vi "autonomous pure pursuit.vi"(10 "Waypoint Data":cluster{"Waypoints":dbl[][], "Reverse?":bool}={"Waypoints"=[[0.0, 0.0], [2.0, 30000.0], [20000.0, 60000.0]], "Reverse?"=FALSE}, 11 "Button":bool) -> ()   [LabVIEW 2018]
uses:
  path data.ctl
  <vilib>/Rock Robotics/WPI/DriverStation/WPI_DriverStationDerivedRobotMode.ctl
  TypeDefs/typedef_enum_Refnums.ctl
  <vilib>/Rock Robotics/WPI/Utilities/WPI_GetSetVariantRefNum.vi
  <vilib>/ptbypt/NI_PtbyPt.lvlib
  <vilib>/Rock Robotics/WPI/RobotDrive/WPI_RobotDriveArcadeDrive_Standard(NoSaturation).vi
  <vilib>/Rock Robotics/Network Tables/NT Write Boolean.vi
panel:
  in  "Path Data":T1={"Path"=[], "Target Velocities"=[], "Robot Location"=[0.0, 0.0], "Relative Robot Angle (rad)"=0.0, "Curvature"=0.0, "Lookahead Point"=[0.0, 0.0], "Lookahead Index"=0.0, "Closest Point"=[0.0, 0.0], "Closest Point Index"=0, "Left Velocity"=0.0, "Right Velocity"=0.0, "Left Encoder Vel"=0, "Right Encoder Vel"=0, "Left Encoder Pos"=0, "Right Encoder Pos"=0, "Inital Robot Angle (deg)"=0.0}
  in  "Diagnostic?":bool=TRUE
  in  "Tuning":T2={"Kv Left"=0.00023, "Kv Right"=0.00023, "Kp Left"=0.0001, "Kp Right"=0.0001}
  out "Loop Time":u32=44680
  out "Exp. Curvature":dbl[](graph)=[0.0, 1.4034333257619034e-07, 3.165606565156983e-07, 5.735690112841907e-07, 9.783335869805837e-07, 1.6388561568734111e-06, 2.7401762932584762e-06, 4.610837725094686e-06, 7.868434900770625e-06, 1.3752057162216792e-05, 2.4965310123263664e-05, 4.7908917652252264e-05, 6.401235309575295e-05, 3.360888592844542e-05, 1.8452253376050564e-05, 1.0514808142316512e-05, 6.145592499109037e-06, 3.650831804118769e-06, 2.191028177213592e-06, 1.3231905148774929e-06, 8.018237673268363e-07, 4.861886501530978e-07, 2.9338742319180646e-07, 1.7372213438406245e-07, 9.640327443482198e-08, 4.0874668672438526e-08, 0.0]
  out "Curvature":dbl(graph)
  out "Target Velocities":cluster{dbl, dbl}(graph)={850.0, 850.0}
  in  "Lookahead Distance":dbl=5000.0 format="%#_13g"
  out "Path":T3(graph)=[{"Smooth Path"=[0.0, 3.9831976339745525, 8.918786774310743, 15.996756278926227, 26.94310215462526, 44.45175679243214, 72.85576199340136, 119.21333672590853, 195.06952147459873, 319.3449114169336, 523.0654465520985, 857.1178508590853, 1404.971654642396, 2303.5684955547395, 3415.918100969553, 4658.468244850319, 5980.216850342943, 7349.961644912561, 8748.499353660785, 10163.825114581763, 11588.130666803412, 13015.85297046767, 14442.283167634836, 15862.389189218296, 17269.55815292861, 18653.942887255045, 20000.0], "Smooth Path"=[0.0, 2604.6593521886216, 5208.4834070465695, 7810.428161388078, 10408.979451847843, 13001.776283234469, 15585.016727668002, 18152.511956181766, 20694.135215630122, 23193.291890529486, 25622.77148689383, 27937.944042539046, 30065.60256829882, 32209.66168633789, 34363.622817575204, 36523.46279208931, 38686.62801955882, 40851.39631476969, 43016.44613594504, 45180.526806154805, 47342.144596973565, 49499.19086028001, 51648.41344856078, 53784.60445996854, 55899.29829439407, 57978.65493411005, 60000.0]}, {"Smooth Path"=[-155.34781165121697, -32.634161371312175], "Smooth Path"=[-10126.308473842537, -2127.2496942088364]}, {"Smooth Path"=[0.0], "Smooth Path"=[0.0]}, {"Smooth Path"=[0.0, -155.34781165121697], "Smooth Path"=[0.0, -10126.308473842537]}]
  in  "Config":T4={"Path"={"Spacing"=2608.0, "Smooth Weight"=0.8, "Tolerance"=0.01}, "Kinematics"={"Max Vel"=850.0, "Max Accel"=200.0, "Curvature Const"=1.0}}
  in  "Track Width":dbl=13000.0 format="%#_13g"
  out "Right Output":dbl=0.24650000000000002
  out "Left Output":dbl=0.23800000000000002
  out "Left Velocity":T5(graph)={"Quadrature Velocity"=0, "Left Velocity"=850.0}
  out "Right Velocity":T6(graph)={"Quadrature Velocity"=0, "Right Velocity"=850.0}
  out "Robot Angle":dbl=-0.87890625
  out "Curvature":dbl
  out "Robot Location":dbl[](array[numeric])=[-155.34781165121697, -10126.308473842537]
  out "Right Velocity":dbl=850.0
  out "Left Velocity":dbl=850.0
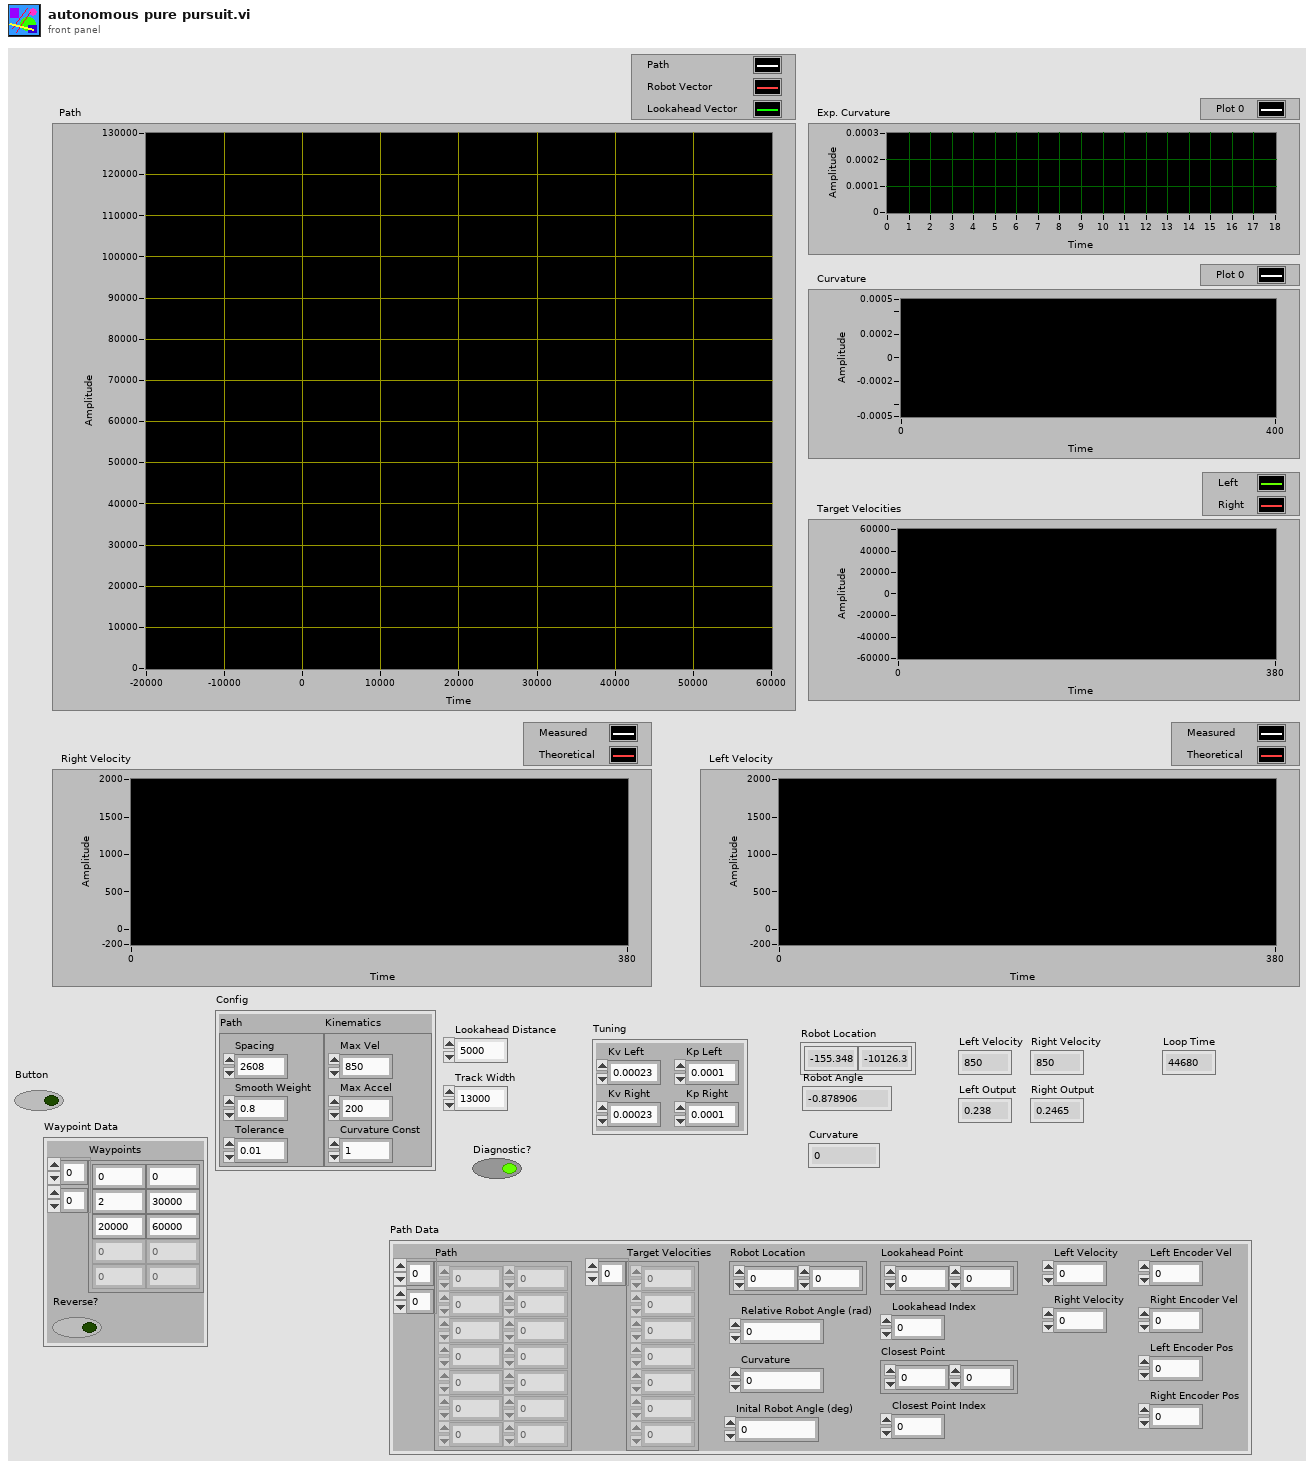
[diagram p1: front panel]
types:
  T1 = typedef "path data.ctl" = cluster{"Path":dbl[][], "Target Velocities":dbl[], "Robot Location":dbl[], "Relative Robot Angle (rad)":dbl, "Curvature":dbl, "Lookahead Point":dbl[], "Lookahead Index":dbl, "Closest Point":dbl[], "Closest Point Index":i32, "Left Velocity":dbl, "Right Velocity":dbl, "Left Encoder Vel":i32, "Right Encoder Vel":i32, "Left Encoder Pos":i32, "Right Encoder Pos":i32, "Inital Robot Angle (deg)":dbl}
  T2 = cluster{"Kv Left":dbl, "Kv Right":dbl, "Kp Left":dbl, "Kp Right":dbl}
  T3 = cluster{"Smooth Path":dbl[], "Smooth Path":dbl[]}[]
  T4 = cluster{"Path":cluster{"Spacing":dbl, "Smooth Weight":dbl, "Tolerance":dbl}, "Kinematics":cluster{"Max Vel":dbl, "Max Accel":dbl, "Curvature Const":dbl}}
  T5 = cluster{"Quadrature Velocity":i32, "Left Velocity":dbl}
  T6 = cluster{"Quadrature Velocity":i32, "Right Velocity":dbl}
  T7 = typedef "WPI_DriverStationDerivedRobotMode.ctl" = enum16{"Init", "Execute", "Stop"}
  T8 = typedef "typedef_enum_Refnums.ctl" = enum16{"Ball_Encoder", "Ball_Motor", "Camera", "Linefollow_3", "Linefollow_2", "Linefollow_1", "Gyro", "Hatch_Solenoid", "Climb_Back_Solenoid", "Arm_Encoder", "Arm_Motor", "Lift_Encoder", "Drive", "Drive_Motor_R", "Drive_Motor_L", "Drive_Encoder_R", "Drive_Encoder_L", "Joy_R", "Joy_L", "Wrist_Motor", "Wrist_Encoder", "Climb Upper Limit", "Climb Lower Limit ", "Climb_Front_Motor"}
  T9 = typedef "Teleop Data Cluster.ctl" = cluster{"Drive Forward Input ":dbl, "Drive Twist Input":dbl, "Drive Output":dbl, "Drivetwist Output":dbl, "Left Joystick Buttons":bool[], "Left Joystick Axis":dbl[], "Right Joystick Axis":dbl[], "Right Joystick Button":bool[], "Arm Encoder":dbl, "Left Drive Encoder":dbl, "Right Drive Encoder":dbl, "Gyro Angle ":dbl, "Arm Joystick Output  ":dbl, "Line Follower L, C, R ":bool[], "Line follow?":bool, " Climb Solenoid":bool, "Wrist Encoder Count":dbl, "Wrist Joystick Output":dbl, "Ball Encoder Count":dbl, "Ball Output":dbl, "Climb Encoder":dbl, "Climb Motor Output":dbl, " Hatch Solenoid":bool, "Arm Setpoint ":dbl, "Wrist Setpoint ":dbl, "Arm Joystick Enabled?":bool, "Wrist Joystick Enabled":bool, "Vision String":string}
  T10 = typedef "WPI_RobotDriveDevRef.ctl" = cluster{"DevStatus":errorcluster, "Motors[]":T11[], "Square Inputs":bool, "Max Output":dbl}
  T11 = typedef "WPI_MotorControlDeviceRef.ctl" = cluster{"DeviceStatus":errorcluster, "Type":T12, "PWM":cluster{"PWM Channel":T13, "DeadBand":T14}, "CAN":cluster{"Device Number":u8, "SetOutput VI Ref":variant, "GetOutput VI Ref":variant, "Enable VI Ref":variant, "Disable VI Ref":variant, "Data":variant}, "Invert":bool, "DIO PWM":cluster{"PWM \"Enable\" Channel":T13, "DIOChannel":T15, "PWM Rate":dbl}}
  T12 = typedef "WPI_MotorControlType.ctl" = enum16{"PWM", "CAN", "DIO PWM"}
  T13 = typedef "FPGA_DIOPWMChannel.ctl" = enum8{"PWM 0", "PWM 1", "PWM 2", "PWM 3", "PWM 4", "PWM 5", "PWM 6", "PWM 7", "PWM 8", "PWM 9", "PWM MXP 0", "PWM MXP 1", "PWM MXP 2", "PWM MXP 3", "PWM MXP 4", "PWM MXP 5", "PWM MXP 6", "PWM MXP 7", "PWM MXP 8", "PWM MXP 9", "Invalid"}
  T14 = typedef "WPI_PWMDeadband.ctl" = cluster{"Name":string, "maxPositivePwm":i32, "minPositivePwm":i32, "centerPwm":i32, "maxNegativePwm":i32, "minNegativePwm":i32, "angularRange":u16}
  T15 = typedef "FPGA_DIOChannel.ctl" = enum8{"DIO 0", "DIO 1", "DIO 2", "DIO 3", "DIO 4", "DIO 5", "DIO 6", "DIO 7", "DIO 8", "DIO 9", "DIO MXP 0", "DIO MXP 1", "DIO MXP 2", "DIO MXP 3", "DIO MXP 4", "DIO MXP 5", "DIO MXP 6", "DIO MXP 7", "DIO MXP 8", "DIO MXP 9", "DIO MXP 10", "DIO MXP 11", "DIO MXP 12", "DIO MXP 13", "DIO MXP 14", "DIO MXP 15", "SPI Port CS1", "SPI Port CS2", "SPI Port CS3", "SPI Port MISO", "SPI Port MOSI", "Invalid"}
  T16 = typedef "CTRE_PigeonIMU_DeviceRef.ctl" = cluster{"DeviceStatus":errorcluster, "Device Number":u8, "Type":T17, "Device ID":u32, "Handle":u64, "UsageFrame":u32, "Library Path":path}
  T17 = typedef "CTRE_PigeonIMU_ConnectionType.ctl" = u32
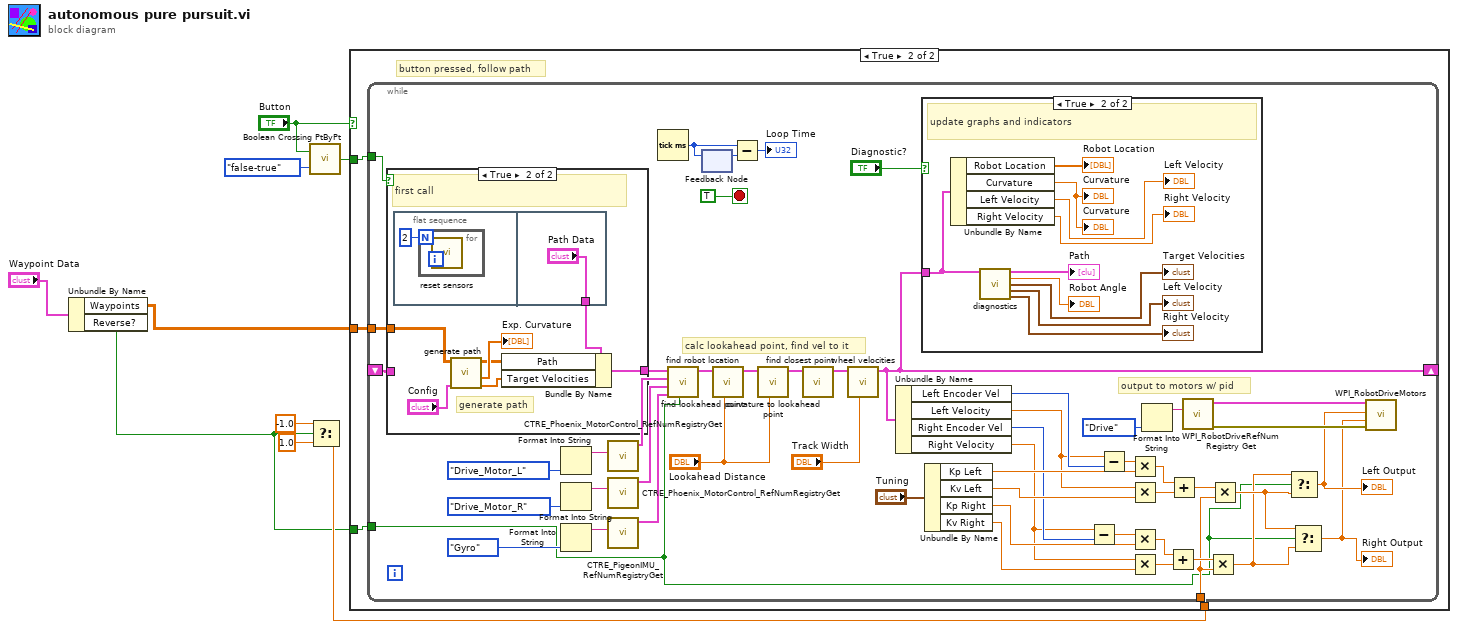
[diagram p0: block diagram]
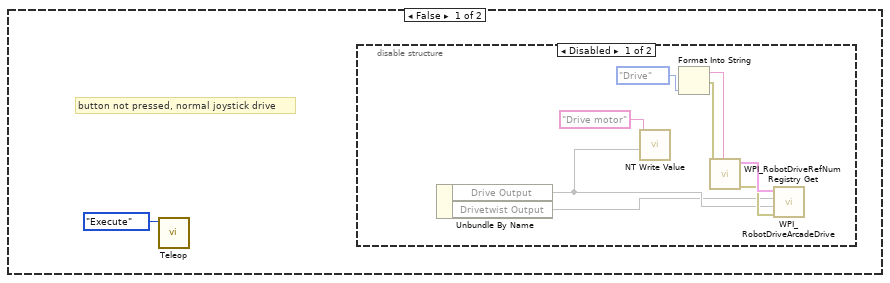
[diagram p2: hidden frame]
diagram:
  n1 = Unbundle By Name("Waypoint Data") -> ("Waypoints"=w2:dbl[][], "Reverse?"=w1:bool)
  n2 = call <vilib>:"Boolean Crossing PtByPt.vi"("direction"=enum16{"either", "false-true", "true-false"}."false-true", "input"="Button") -> ("crossing"=w7:bool)  [unwired: 1 in]
  n3 = Select(t=-1.0, s=w1, f=1.0) -> (s? t:f=w4:dbl)
  n4 = case shown="True" "Button" {
    tunnel: w7 -> [_ w23]
    tunnel: w4 -> [_ w22]
    tunnel: w1 -> [_ w21]
    tunnel: w2 -> [_ w20]
    frame False {
      # "button not pressed, normal joystick drive"
      n5 = call "Teleop.vi"("Call Context"=WPI_DriverStationDerivedRobotMode."Execute") -> ()  [unwired: 11 in]
      n6 = disable-structure shown="Disabled" {
        frame Disabled {
          n7 = Unbundle By Name() -> (w13:T9, "Drive Output"=w14, "Drivetwist Output"=w11)
          n8 = call-poly <vilib>:"NT Write Value.vi"("Boolean"=w14, "Name"="Drive motor") -> ()  [unwired: 9 in, 1 out]
          n9 = Format Into String(typedef_enum_Refnums."Drive" ("RefNums")) -> (resulting string=w18:string, error out=w16:errorcluster)  [unwired: 3 in]
          n10 = call <vilib>:"WPI_RobotDriveRefNum Registry Get.vi"("error in (no error)"=w16, "refnum name"=w18) -> ("error out"=w15:errorcluster, "RobotDriveDevRef"=w19:T10)  [unwired: 8 in]
          n11 = call-poly <vilib>:"WPI_RobotDriveArcadeDrive.vi"("error in (no error)"=w15, "Y axis value"=w14, "X axis value"=w11, "RobotDriveDevRef"=w19) -> ()  [unwired: 5 in, 3 out]
        }
        frame Enabled {
        }
      }
    }
    frame True {
      # "button pressed, follow path"
      n12 = while {
        tunnel: w23 -> [w39]
        shift-right: [w41] -> _
        shift-left: _ -> [w50]
        tunnel: w22 -> [w30]
        tunnel: w21 -> [w25]
        tunnel: w20 -> [w24]
        stop <- TRUE stop-if-true
        # "calc lookahead point, find vel to it"
        # "output to motors w/ pid"
        n13 = case shown="True" w39 {
          tunnel: [w86 w89] -> w40
          tunnel: w50 -> [w86 _]
          tunnel: w24 -> [_ w88]
          frame False {
          }
          frame True {
            # "generate path"
            # "first call"
            n14 = flat-sequence {
              tunnel: ["Path Data"] -> w87
              frame #0 {
                n15 = for {
                  N: 2 -> [_]
                  n16 = call "reset sensors.vi"() -> ()  [unwired: 12 in]
                }
              }
              frame #1 {
              }
            }
            n17 = call "generate path.vi"("Config"="Config", "Waypoints"=w88) -> ("Target Velocities"=w90:dbl[], "Curvatures"=→"Exp. Curvature":dbl[], "Smooth Path"=w91:dbl[][])  [unwired: 4 in, 3 out]
            n18 = Bundle By Name(cluster=w87, "Path"=w91, "Target Velocities"=w90) -> (w89:T1)
          }
        }
        n19 = Format Into String(typedef_enum_Refnums."Drive_Motor_L" ("RefNums")) -> (resulting string=w35:string)  [unwired: 3 in, 1 out]
        n20 = Format Into String(typedef_enum_Refnums."Drive_Motor_R" ("RefNums")) -> (resulting string=w34:string)  [unwired: 3 in, 1 out]
        n21 = Format Into String(typedef_enum_Refnums."Gyro" ("RefNums")) -> (resulting string=w33:string)  [unwired: 3 in, 1 out]
        n22 = call <vilib>:"CTRE_Phoenix_MotorControl_RefNumRegistryGet.vi"("refnum name"=w35) -> ("PhoenixMotorControlDevRef"=w46:T11)  [unwired: 9 in, 1 out]
        n23 = call <vilib>:"CTRE_Phoenix_MotorControl_RefNumRegistryGet.vi"("refnum name"=w34) -> ("PhoenixMotorControlDevRef"=w47:T11)  [unwired: 9 in, 1 out]
        n24 = call <vilib>:"CTRE_PigeonIMU_RefNumRegistryGet.vi"("refnum name"=w33) -> ("PigeonIMUDevRef"=w48:T16)  [unwired: 9 in, 1 out]
        n25 = Tick Count (ms)() -> (millisecond timer value=w67:u32)
        n26 = call "find robot location.vi"("Reverse?"=w25, "Pigeon Reference"=w48, "Right Encoder Reference"=w47, "Left Encoder Reference"=w46, "Path Data"=w40) -> ("Path Data"=w49:T1)  [unwired: 6 in]
        n27 = feedback-in #1(w67) -> ()
        n28 = feedback #1() -> (w66:u32)  [unwired: 1 in]
        n29 = call "find lookahead point.vi"("Lookahead Distance"="Lookahead Distance", "Path Data"=w49) -> ("Path Data"=w53:T1)  [unwired: 9 in]
        n30 = Subtract(x=w67, y=w66) -> (x-y=→"Loop Time":u32)
        n31 = call "curvature to lookahead point.vi"("Lookahead Distance"="Lookahead Distance", "Path Data"=w53) -> ("Path Data"=w52:T1)  [unwired: 9 in]
        n32 = call "find closest point.vi"("Path Data"=w52) -> ("Path Data"=w51:T1)  [unwired: 10 in]
        n33 = call "wheel velocities.vi"("Track Width"="Track Width", "Path Data"=w51) -> ("Path Data"=w41:T1)  [unwired: 9 in]
        n34 = Unbundle By Name(w41) -> ("Left Encoder Vel"=w45:i32, "Left Velocity"=w44:dbl, "Right Encoder Vel"=w43:i32, "Right Velocity"=w42:dbl)
        n35 = case shown="True" "Diagnostic?" {
          tunnel: w41 -> [_ w76]
          frame False {
          }
          frame True {
            # "update graphs and indicators"
            n36 = Unbundle By Name(w76) -> ("Robot Location"=→"Robot Location":dbl[], "Curvature"=→"Curvature" →"Curvature":dbl, "Left Velocity"=→"Left Velocity":dbl, "Right Velocity"=→"Right Velocity":dbl)
            n37 = call "diagnostics.vi"("Path Data"=w76) -> ("Path"=→"Path":T3, "Robot Angle (deg)"=→"Robot Angle":dbl, "Target Velocities"=→"Target Velocities":cluster{dbl, dbl}, "Left Velocity"=→"Left Velocity":T5, "Right Velocity"=→"Right Velocity":T6)  [unwired: 10 in]
          }
        }
        n38 = Unbundle By Name("Tuning") -> ("Kp Left"=w61:dbl, "Kv Left"=w60:dbl, "Kp Right"=w59:dbl, "Kv Right"=w58:dbl)
        n39 = Subtract(x=w42, y=w43) -> (x-y=w69:dbl)
        n40 = Subtract(x=w44, y=w45) -> (x-y=w71:dbl)
        n41 = Multiply(x=w71, y=w61) -> (x*y=w70:dbl)
        n42 = Multiply(x=w44, y=w60) -> (x*y=w73:dbl)
        n43 = Multiply(x=w69, y=w59) -> (x*y=w68:dbl)
        n44 = Multiply(x=w42, y=w58) -> (x*y=w72:dbl)
        n45 = Format Into String(typedef_enum_Refnums."Drive" ("RefNums")) -> (resulting string=w31:string)  [unwired: 3 in, 1 out]
        n46 = Add(x=w68, y=w72) -> (x+y=w64:dbl)
        n47 = Add(x=w70, y=w73) -> (x+y=w63:dbl)
        n48 = call <vilib>:"WPI_RobotDriveRefNum Registry Get.vi"("refnum name"=w31) -> ("error out"=w55:errorcluster, "RobotDriveDevRef"=w54:T10)  [unwired: 9 in]
        n49 = Multiply(x=w64, y=w30) -> (x*y=w26:dbl)
        n50 = Multiply(x=w63, y=w30) -> (x*y=w27:dbl)
        n51 = Select(t=w26, s=w25, f=w27) -> (s? t:f=w29:dbl)
        "Left Output" <- w29
        n52 = Select(t=w27, s=w25, f=w26) -> (s? t:f=w28:dbl)
        "Right Output" <- w28
        n53 = call <vilib>:"WPI_RobotDriveMotors.vi"("error in (no error)"=w55, "RightSpeed"=w28, "LeftSpeed"=w29, "RobotDriveDevRef"=w54) -> ()  [unwired: 5 in, 3 out]
      }
    }
  }
